vi "Scratch_plant.vi"() -> ()   [LabVIEW 2016]
uses:
  <vilib>/xnet/xnet.llb/XNET Read (Signal Single-point).vi
panel:
  in  "stop":bool
  out "data":dbl[](array[numeric]) format="%.2f"
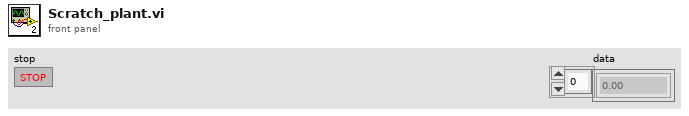
[diagram p1: front panel]
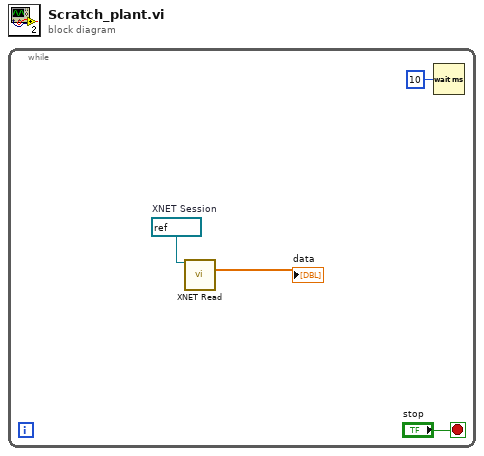
[diagram p0: block diagram]
diagram:
  n1 = while {
    stop <- "stop" stop-if-true
    w4 = refnum<k21> "Test"  # XNET Session
    n2 = call-poly <vilib>:"XNET Read.vi"("session in"=w4) -> ("data"=→"data":dbl[])  [unwired: 12 in, 2 out]
    n3 = Wait (ms)(milliseconds to wait=u32 10) -> ()  [unwired: 1 out]
  }
